vi "Main Loop.vi"(8 "error in (no error)":errorcluster, 10 "Chart Notifier":refnum<notifier>, 11 "Message Queues":T1) -> (0 "error out":errorcluster)   [LabVIEW 2018, in "Agitator Module.lvlib" / "Agitator Module Engine.lvlib"]
uses:
  Agitator Module Engine.lvlib
  Agitator Message Queues.ctl
  support/Message Queue/Message Cluster.ctl
  Feed Module/Controls/Agitator Module Display.ctl
  Feed Module/Controls/Agitator Module State Cluster.ctl
  Pump Module Folder/Measure Instrument/State Enum.ctl
  Feed Module/Controls/Agitator Module Config Cluster.ctl
  <vilib>/Utility/miscctls.llb/LVPoint32TypeDef.ctl
  Feed Module/Controls/Agitator Module Settings Cluster.ctl
  IKA EUROSTAR/IKA EUROSTAR Settings.ctl
  <vilib>/Platform/TimedLoop/XDataNode/timing_clust.ctl
  <vilib>/Platform/TimedLoop/XDataNode/nitl_modes.ctl
  <vilib>/Platform/TimedLoop/XDataNode/wakeup.ctl
  Tag VIs/Tag FGV Operation Enum.ctl
  support/Message Queue/Enqueue Message (Single).vi
  <vilib>/Platform/TimedLoop/XDataNode/XDataNode.xnode
  support/Message Queue/Message Queue.lvlib
  <vilib>/Platform/TimedLoop/XDataNode/XDNodeRunTimeDep.lvlib
  Agitator Module.lvlib
  Shared Variables/Dynamic Shared Variables.lvlib
  support/Support Library.lvlib
  Pump Module Folder/Measure Instrument/Pump Module Engine.lvlib
  IKA EUROSTAR/IKA EUROSTAR.lvlib
panel:
  out "Period (s) 2":dbl format="%_4g"
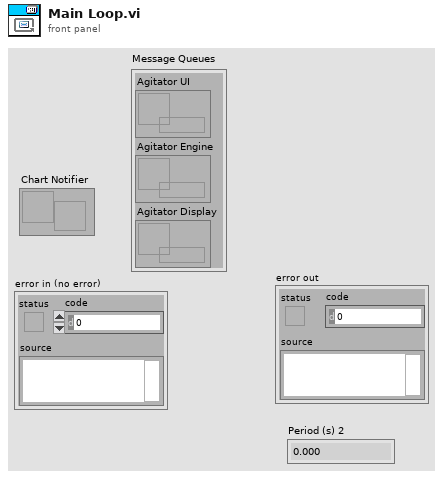
[diagram p1: front panel]
types:
  T1 = typedef "Agitator Module.lvlib/Agitator Message Queues.ctl" = cluster{"Agitator UI":refnum<queue>, "Agitator Engine":refnum<queue>, "Agitator Display":refnum<queue>}
  T2 = typedef "XDNodeRunTimeDep.lvlib/timing_clust.ctl" = cluster{"Expected End [f-1]":u64, "Actual End [f-1]":u64, "Finished Late? [f-1]":bool, "Expected End [i-1]":u64, "Actual End [i-1]":u64, "Finished Late? [i-1]":bool, "Expected Start [i]":u64, "Actual Start [i]":u64, "Expected Start [f]":u64, "Actual Start [f]":u64, "Source Name":string, "Structure Name":string, "Period":i64, "Deadline":i64, "Offset":i64, "Start":i64, "Priority":i32, "Timeout":i32, "Mode":T3, "Wakeup Reason":T4, "Error":errorcluster, "Source Type":string, "Secondary Source Type":string, "Global End Time":u64, "Global Start Time":u64, "Frame Duration":u64, "Iteration Duration":u64, "Assigned CPU":i32, "I/O Scan Engine Mode":u32}
  T3 = typedef "XDNodeRunTimeDep.lvlib/nitl_modes.ctl" = enum32{"No Change", "Process missed periods, maintain original phase", "Discard missed periods, maintain original phase", "Process missed periods, ignore original phase", "Discard missed periods, ignore original phase"}
  T4 = typedef "XDNodeRunTimeDep.lvlib/wakeup.ctl" = enum32{"Normal", "Aborted", "Asynchronous wakeup", "Timing source error", "Timed loop error", "Timeout"}
  T5 = cluster{"enable? (F)":bool, "name":string, "alarm on":bool, "priority":u32, "ack type":enum16{"Auto", "User", "None", "Each Occurrence"}, "area":string, "description":string, "log? (T)":bool}
  T6 = typedef "Tag FGV Operation Enum.ctl" = enum16{"Init", "Set Notification Queue", "Create Tag", "Commit", "Write Tag (Numeric)", "Write Tag (Boolean)", "Read All Tags", "Read One Tag", "Delete Tag Category", "Set Alarm Parameters (Numeric)", "Set Alarm Parameters (Boolean)", "Enable All Alarms", "Disable All Alarms", "Delete All Tags", "Read Alarms", "Ack Alarm", "Read Alarm Parameters (Numeric)", "Read Alarm Parameters (Boolean)"}
  T7 = enum32{"u32BitField", "bool", "double", "string", "int8", "uint8", "int16", "uint16", "int32", "uint32", "int64", "uint64", "single", "double waveform", "int16 waveform", "array of boolean", "array of int8", "array of uint8", "array of int16", "array of uint16", "array of int32", "array of uint32", "array of int64", "array of uint64", "array of single", "array of double", "array of double waveform", "array of int16 waveform", "array of string", "variant", "timestamp", "fixed point", "custom"}
  T8 = typedef "Pump Module.lvlib/Pump Module Engine.lvlib/State Enum.ctl" = enum16{"Measuring", "Idle", "Paused"}
  T9 = typedef "Agitator Module.lvlib/Agitator Module Config Cluster.ctl" = cluster{"GUID":string, "Drop Coords":T10, "Process Name":string, "User name":string, "Queue Name":string, "Settings":T11, "Load Count":i32}
  T10 = typedef "LVPoint32TypeDef.ctl" = cluster{"Horizontal":i32, "Vertical":i32}
  T11 = typedef "Agitator Module.lvlib/Agitator Module Settings Cluster.ctl" = cluster{"Cycle Period":dbl, "Agitator Type":string, "Setpoint (µm)":dbl, "IKA EUROSTAR Settings":T12}
  T12 = typedef "IKA EUROSTAR.lvlib/IKA EUROSTAR Settings.ctl" = cluster{"VISA resource name":refnum<visa-resource-name>, "Simulated?":bool}
  T13 = typedef "Agitator Module.lvlib/Agitator Module State Cluster.ctl" = cluster{"State":T8, "Start Time":timestamp, "Current Time":timestamp, "Agitator Module Config":T9, "Output Error":bool, "Log Started":bool, "First Iteration":bool, "Data":cluster{"Agitator rpm Value":dbl}, "Agitator On?":enum16{"Off", "On", "Not Initialized", "Over Cutoff"}}
  T14 = typedef "Agitator Module.lvlib/Agitator Module Display.ctl" = cluster{"Agitator On?":enum16{"Off", "On", "Not Initialized", "Over Cutoff"}, "Agitator RPM Value":dbl, "Cycle Period":dbl}
  T15 = enum16{"Off", "On", "Not Initialized", "Over Cutoff"}
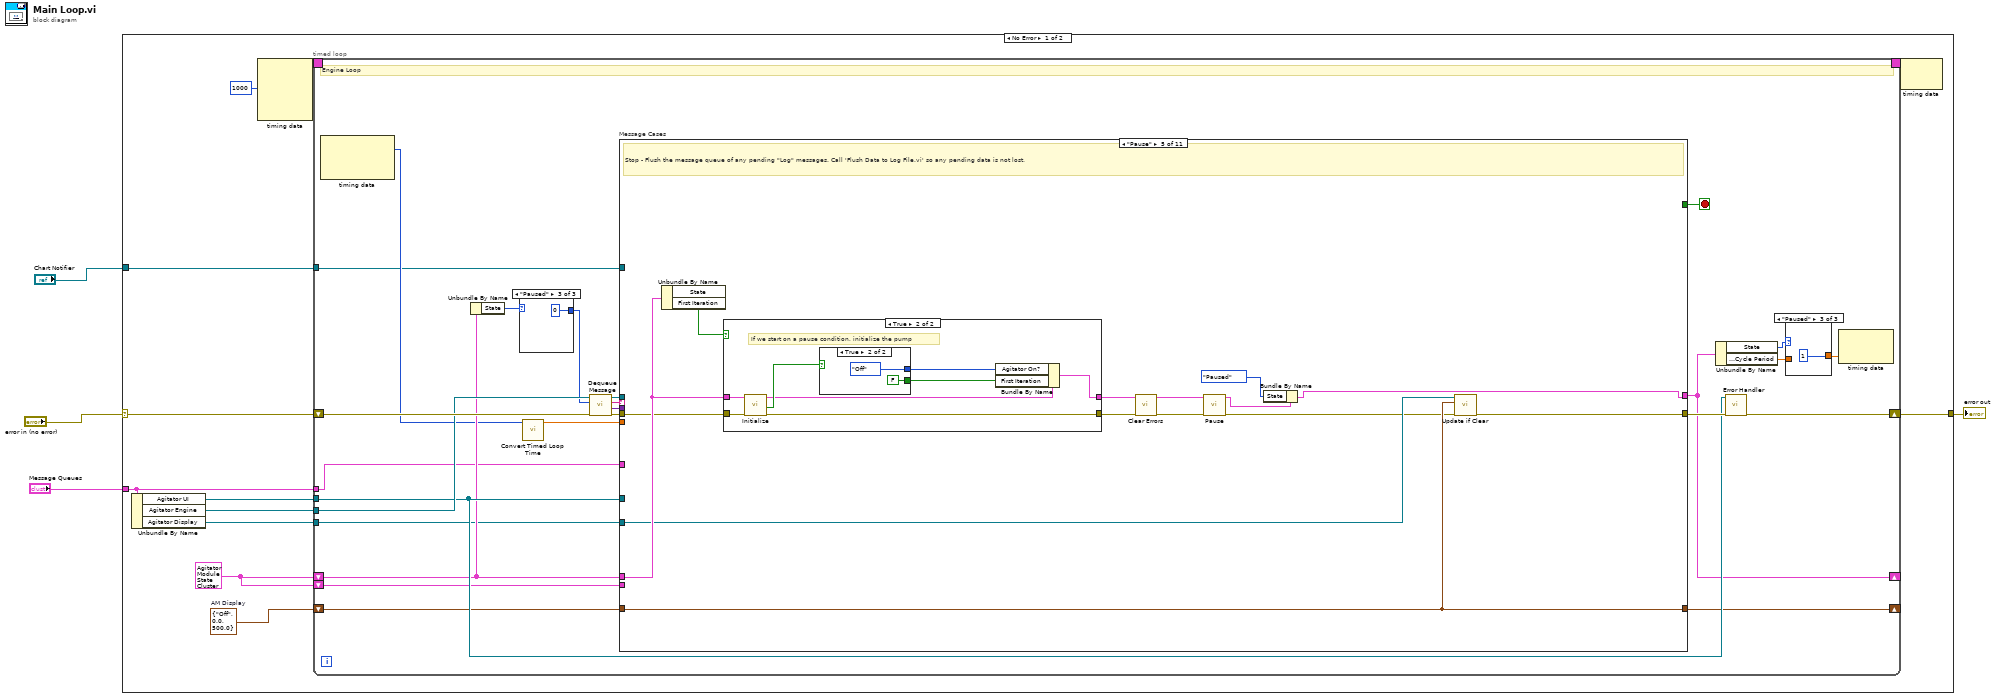
[diagram p0: block diagram]
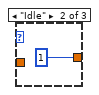
[diagram p3: hidden frame]
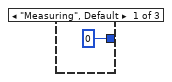
[diagram p4: hidden frame]
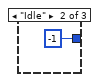
[diagram p5: hidden frame]
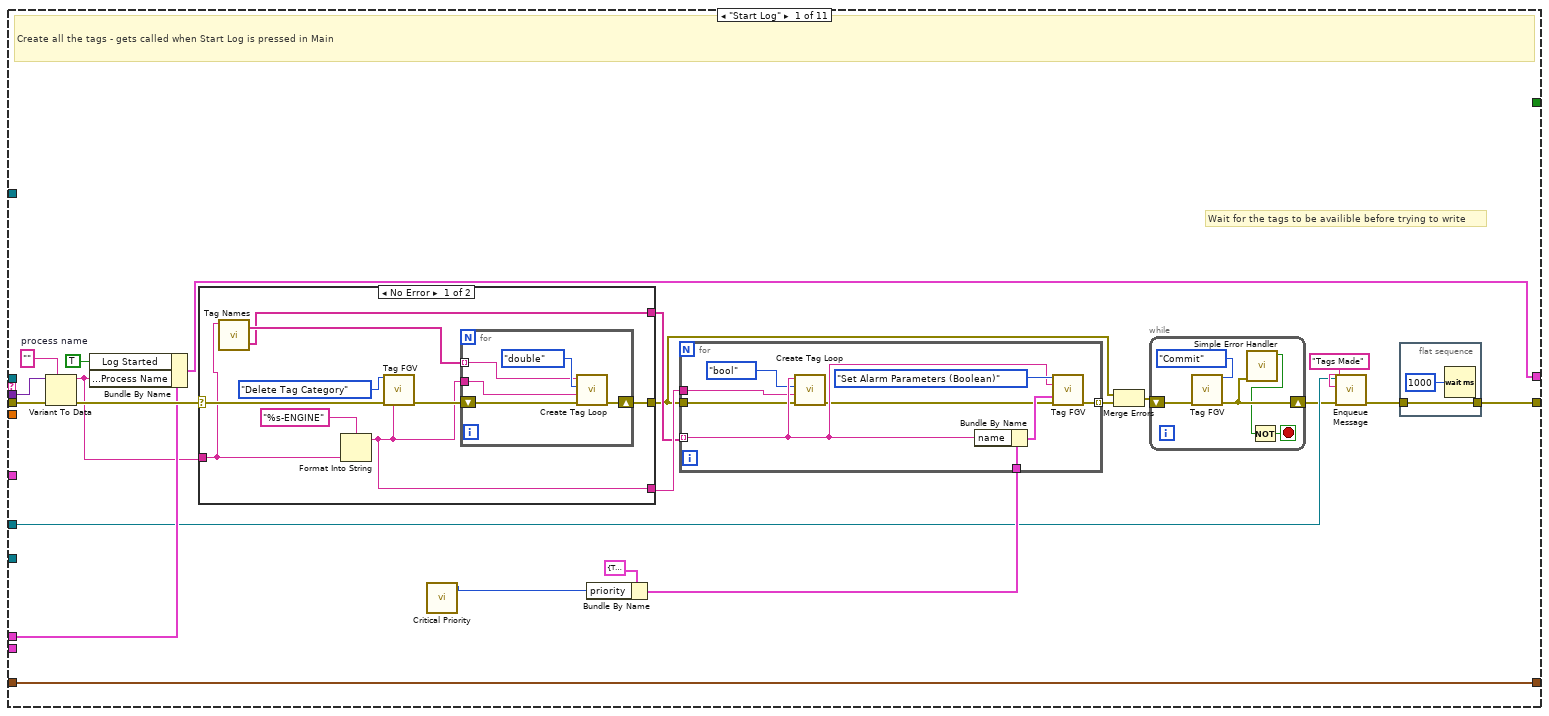
[diagram p6: hidden frame]
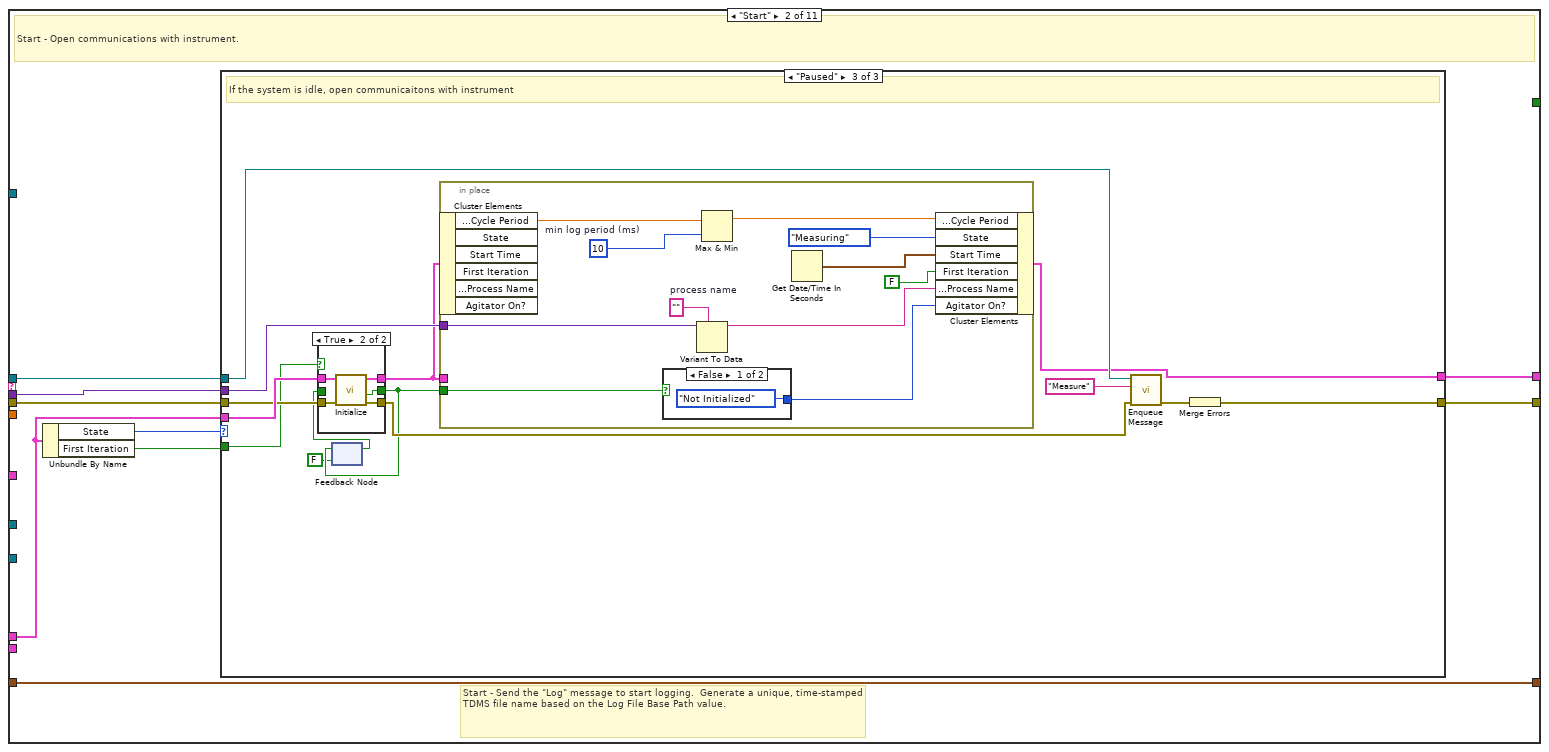
[diagram p8: hidden frame]
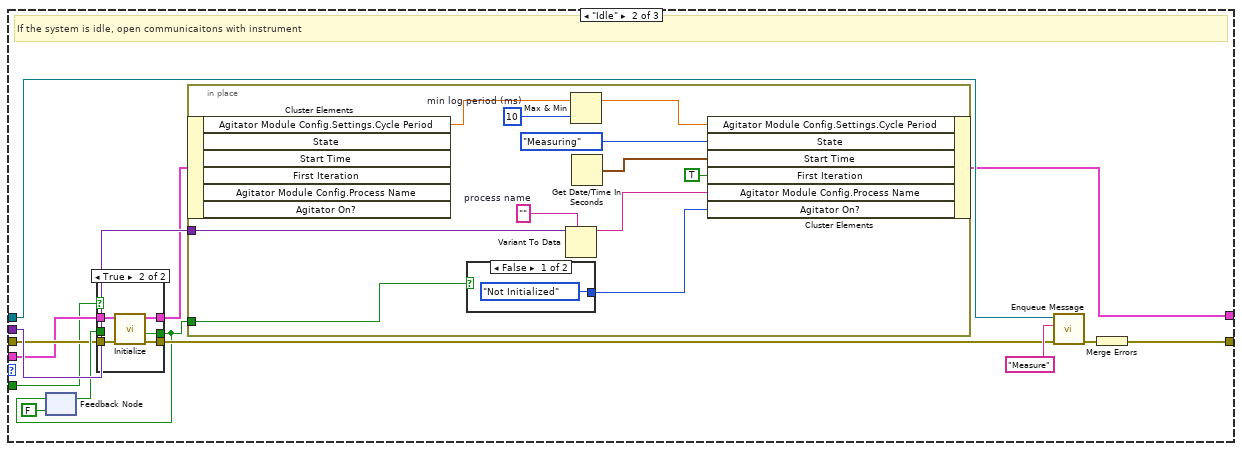
[diagram p10: hidden frame]
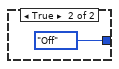
[diagram p11: hidden frame]
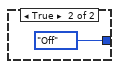
[diagram p13: hidden frame]
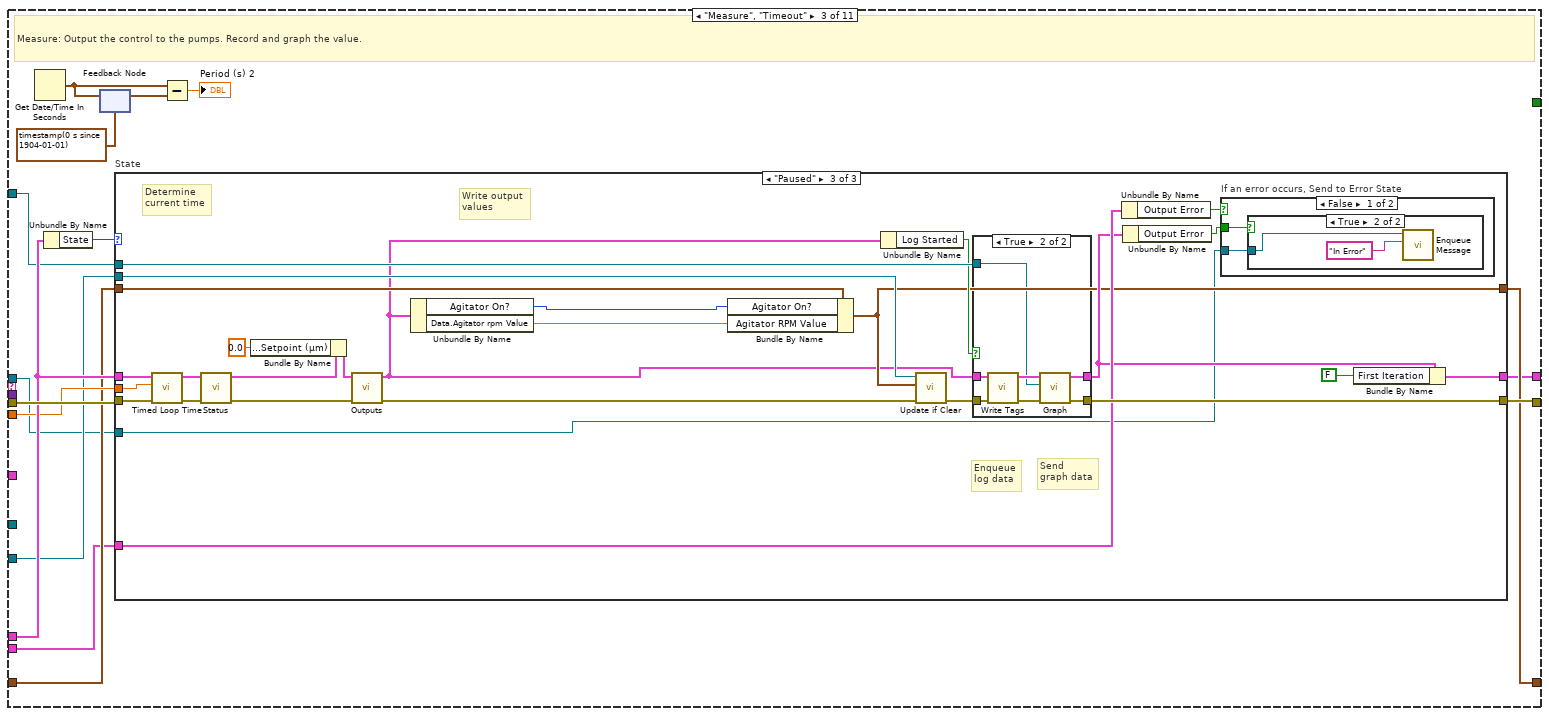
[diagram p15: hidden frame]
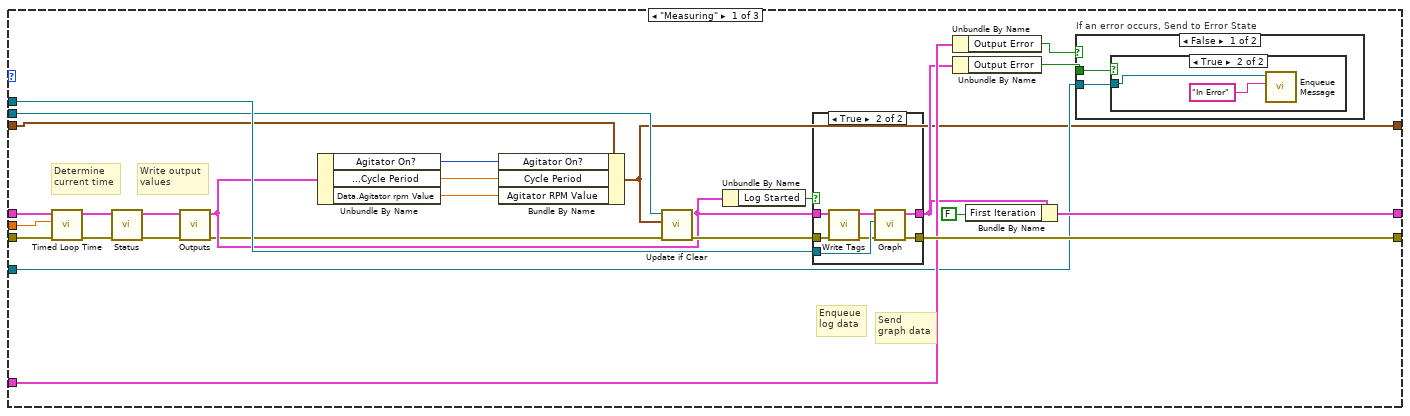
[diagram p16: hidden frame]
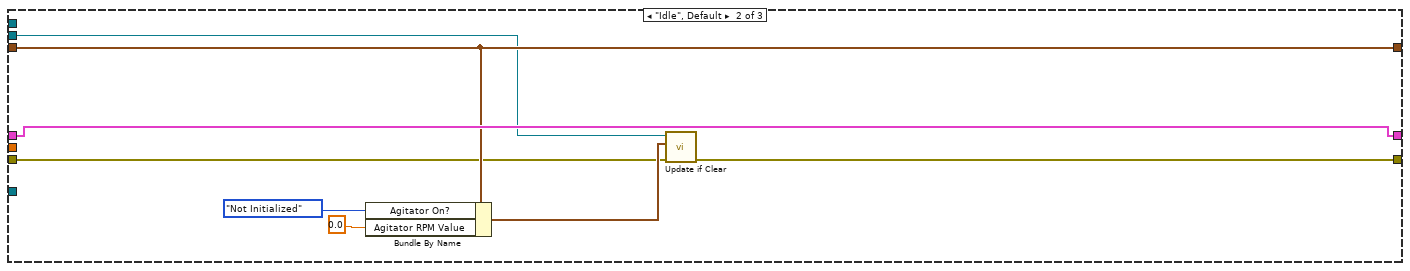
[diagram p20: hidden frame]
diagram:
  n1 = case shown="No Error" "error in (no error)" {
    selector: "error in (no error)" -> [w15 w405]
    tunnel: "Message Queues" -> [w11 _]
    tunnel: [w16 w405] -> w4
    tunnel: "Chart Notifier" -> [w9 _]
    frame No Error {
      w5 = T13 {"State"=enum."Idle", "Start Time"=timestamp(0 s since 1904-01-01), "Current Time"=timestamp(0 s since 1904-01-01), "Agitator Module Config"={"GUID"="", "Drop Coords"={"Horizontal"=0, "Vertical"=0}, "Process Name"="", "User name"="", "Queue Name"="", "Settings"={"Cycle Period"=500.0, "Agitator Type"="", "Setpoint (µm)"=0.0, "IKA EUROSTAR Settings"={"VISA resource name"="", "Simulated?"=FALSE}}, "Load Count"=0}, "Output Error"=FALSE, "Log Started"=FALSE, "First Iteration"=FALSE, "Data"={"Agitator rpm Value"=0.0}, "Agitator On?"=enum."Off"} ("Sonicator Module State Cluster")
      w6 = T14 {"Agitator On?"=enum."Off", "Agitator RPM Value"=0.0, "Cycle Period"=500.0}  # AM Display
      n2 = Unbundle By Name(w11) -> ("Agitator UI"=w14:refnum<queue>, "Agitator Engine"=w10:refnum<queue>, "Agitator Display"=w8:refnum<queue>)
      n3 = node-c288(i64 1000 ("Period")) -> (w13:T2)  [unwired: 3 in]
      n4 = timed-loop {
        tunnel: w10 -> [w35]
        shift-right: [w17] -> _
        shift-left: w5 -> [w31]
        shift-right: [w33] -> w16
        shift-left: w15 -> [w40]
        tunnel: w14 -> [w32]
        timing: w13 -> [_]
        timing-out: [_] -> w12
        tunnel: w11 -> [w23]
        tunnel: w9 -> [w22]
        tunnel: w8 -> [w21]
        shift-right: [w20] -> _
        shift-left: w6 -> [w19]
        shift-left: w5 -> [w18]
        stop <- w41 stop-if-true
        # "Engine Loop"
        n5 = node-c288() -> (w25:i64)  [unwired: 1 in, 2 out]
        n6 = Unbundle By Name(w31) -> ("State"=w30:T8)
        n7 = case shown="\"Paused\"" w30 {
          tunnel: [0 ("timeout in ms (-1)") -1 ("timeout in ms (-1)") 0 ("timeout in ms (-1)")] -> w29
          frame "Measuring", Default {
          }
          frame "Idle" {
          }
          frame "Paused" {
          }
        }
        n8 = call "Convert Timed Loop Time.vi"("Actual Start [i]"=w25) -> ("ET since start (s)"=w24:dbl)  [unwired: 10 in]
        n9 = call "Dequeue Message.vi"("error in (no error)"=w40, "timeout in ms (-1)"=w29, "Message Queue"=w35) -> ("error out"=w39:errorcluster, "Message Data"=w37:variant, "Message"=w38:string, "dup Message Queue"=w36:refnum<queue>)  [unwired: 5 in]
        n10 = case "Message Cases" shown="\"Pause\"" w38 {
          selector: w38 -> [_ _ _ _ _ _ _ _ _ _ w394]
          tunnel: w36 -> [_ w113 w190 _ _ _ w349 _ w368 _ _]
          tunnel: w39 -> [w59 w112 w200 w295 w321 w343 w352 w359 w363 w392 _]
          tunnel: [w55 w114 w201 w290 w318 w340 w354 w358 w373 w391 w393] -> w34
          tunnel: w31 -> [w64 w109 w199 w297 w322 w341 w345 w356 w364 w389 w399]
          tunnel: [w53 w106 w188 w296 w311 w339 w345 w356 w374 w387 w399] -> w17
          tunnel: [_ _ _ _ _ _ TRUE _ _ _ _] -> w41
          tunnel: w37 -> [w73 w110 _ _ _ w344 _ _ _ _ _]
          tunnel: w32 -> [w61 _ _ w299 _ _ w353 _ _ _ _]
          tunnel: w24 -> [_ _ w198 _ _ _ _ _ _ _ _]
          tunnel: w23 -> [_ _ _ _ _ _ _ _ _ _ _]
          tunnel: w22 -> [_ _ w194 _ _ _ _ _ _ _ _]
          tunnel: w21 -> [_ _ w193 w293 w320 _ _ _ w367 _ _]
          tunnel: w19 -> [w74 w108 w192 w292 w319 w342 w346 w357 w372 w390 w400]
          tunnel: [w74 w108 w191 w292 w319 w342 w346 w357 w366 w390 w400] -> w20
          tunnel: w18 -> [_ _ w189 _ _ _ _ _ _ _ _]
          frame "Start Log" {
            w72 = ""  # process name
            # "Wait for the tags to be availible before trying to write"
            # "Create all the tags - gets called when Start Log is pressed in Main"
            n11 = Variant To Data(error in=w59, type=w72, Variant=w73) -> (data=w60:string, error out=w71:errorcluster)
            n12 = Bundle By Name(cluster=w64, "Log Started"=TRUE, "Agitator Module Config.Process Name"=w60) -> (w53:T13)
            n13 = case shown="No Error" w71 {
              selector: w71 -> [w96 w105]
              tunnel: [w99 w105] -> w54
              tunnel: [w94 _] -> w67
              tunnel: [w92 _] -> w66
              tunnel: w60 -> [w91 _]
              frame No Error {
                n14 = call "Tag Names.vi"("Process Name"=w91) -> ("All Boolean Tags"=w92:string[], "All  Numeric Tags"=w93:string[])  [unwired: 8 in, 1 out]
                n15 = Format Into String(format string="%s-ENGINE", w91) -> (resulting string=w94:string)  [unwired: 2 in, 1 out]
                n16 = call "Tag FGV.vi"("Operation"=Tag_FGV_Operation_Enum."Delete Tag Category", "error in (no error)"=w96, "Tag Category"=w94) -> ("error out"=w95:errorcluster)  [unwired: 5 in, 7 out]
                n17 = for {
                  shift-right: [w100] -> w99
                  shift-left: w95 -> [w101]
                  tunnel: w94 -> [w102]
                  tunnel: w93 -> [w103] mode=indexing
                  n18 = call "Create Tag Loop.vi"("error in (no error)"=w101, "Tag Category"=w102, "data type"=T7."double", "Tag Name"=w103) -> ("error out"=w100:errorcluster)  [unwired: 7 in]
                }
              }
              frame Error {
              }
            }
            n19 = call "Critical Priority.vi"() -> ("critical priority"=w70:i32)  [unwired: 11 in]
            n20 = Bundle By Name(cluster=T5 {"enable? (F)"=TRUE, "name"="Boolean", "alarm on"=TRUE, "priority"=1, "ack type"=enum."Each Occurrence", "area"="a", "description"="", "log? (T)"=TRUE} ("Boolean alarm settings"), "priority"=w70) -> (w68:T5)
            n21 = for {
              tunnel: w68 -> [w90]
              tunnel: [w89] -> w65 mode=indexing
              tunnel: w66 -> [w86] mode=indexing
              tunnel: w54 -> [w83]
              tunnel: w67 -> [w84]
              n22 = call "Create Tag Loop.vi"("error in (no error)"=w83, "Tag Category"=w84, "data type"=T7."bool", "Tag Name"=w86) -> ("error out"=w82:errorcluster)  [unwired: 7 in]
              n23 = Bundle By Name(cluster=w90, "name"=w86) -> (w88:T5)
              n24 = call "Tag FGV.vi"("Operation"=Tag_FGV_Operation_Enum."Set Alarm Parameters (Boolean)", "Tag Name"=w86, "Data"=w88, "error in (no error)"=w82) -> ("error out"=w89:errorcluster)  [unwired: 4 in, 7 out]
            }
            n25 = Merge Errors(w54, w65) -> (w58:errorcluster)
            n26 = while {
              shift-right: [w79] -> w57
              shift-left: w58 -> [w80]
              stop <- w77 stop-if-true
              n27 = call "Tag FGV.vi"("Operation"=Tag_FGV_Operation_Enum."Commit", "error in (no error)"=w80) -> ("error out"=w79:errorcluster)  [unwired: 6 in, 7 out]
              n28 = call <vilib>:"Simple Error Handler.vi"("error in (no error)"=w79) -> ("error?"=w78:bool)  [unwired: 4 in, 4 out]
              n29 = Not(x=w78) -> (.not. x?=w77:bool)
            }
            n30 = call-poly "Enqueue Message.vi"("error in (no error)"=w57, "Message"="Tags Made", "Message Queue"=w61) -> ("error out"=w56:errorcluster)  [unwired: 7 in, 1 out]
            n31 = flat-sequence {
              tunnel: [w75] -> w55
              tunnel: w56 -> [w75]
              frame #0 {
                n32 = Wait (ms)(milliseconds to wait=u32 1000) -> ()  [unwired: 1 out]
              }
            }
          }
          frame "Start" {
            # "Start - Send the \"Log\" message to start logging.  Generate a unique, time-stamped TDMS file name based on the Log File Base Path value."
            # "Start - Open communications with instrument."
            n33 = Unbundle By Name(w109) -> ("State"=w111:T8, "First Iteration"=w107:bool)
            n34 = case shown="\"Paused\"" w111 {
              tunnel: [w115 w130 w165] -> w114
              tunnel: w113 -> [_ w127 w162]
              tunnel: w112 -> [w115 w124 w159]
              tunnel: w109 -> [w116 w123 w160]
              tunnel: [w116 w118 w153] -> w106
              tunnel: w110 -> [_ w126 w161]
              tunnel: w107 -> [_ w120 w155]
              frame "Measuring", Default {
                # "The system is already running. Ignore the \"Start\" message."
              }
              frame "Idle" {
                # "If the system is idle, open communicaitons with instrument"
                n35 = feedback #1(FALSE ("Initialized")) -> (w125:bool)
                n36 = case shown="True" w120 {
                  tunnel: w124 -> [w146 w147]
                  tunnel: w123 -> [w144 w148]
                  tunnel: [w144 w151] -> w119
                  tunnel: [w146 w150] -> w122
                  tunnel: [w145 w149] -> w121
                  tunnel: w125 -> [w145 _]
                  frame False {
                  }
                  frame True {
                    n37 = call "Initialize.vi"("error in (no error)"=w147, "Agitator Module State Cluster"=w148) -> ("error out"=w150:errorcluster, "Initialized"=w149:bool, "Agitator Module State Cluster"=w151:T13)  [unwired: 7 in]
                  }
                }
                n38 = feedback-in #1(w121) -> ()
                n39 = in-place {
                  in-place-border: w126 -> [w139]
                  in-place-border: w121 -> [w138]
                  w140 = ""  # process name
                  w141 = 10  # min log period (ms)
                  n40 = in-place-cluster #2(w119) -> ("Agitator Module Config.Settings.Cycle Period"=w137:dbl)  [unwired: 5 out]
                  n41 = case shown="False" w138 {
                    tunnel: [enum16{"Off", "On", "Not Initialized"}."Not Initialized" ("Pump On?") enum16{"Off", "On", "Not Initialized"}."Off" ("Pump On?")] -> w131
                    frame False {
                    }
                    frame True {
                    }
                  }
                  n42 = Variant To Data(type=w140, Variant=w139) -> (data=w132:string)  [unwired: 1 in, 1 out]
                  n43 = Max & Min(x=w137, y=w141) -> (max(x,y)=w136:dbl)  [unwired: 1 out]
                  n44 = Get Date/Time In Seconds() -> (seconds since 1Jan1904=w134:timestamp)
                  n45 = in-place-cluster #2("Agitator Module Config.Settings.Cycle Period"=w136, "State"=State_Enum."Measuring", "Start Time"=w134, "First Iteration"=TRUE, "Agitator Module Config.Process Name"=w132, "Agitator On?"=w131) -> (w118:T13)
                }
                n46 = call-poly "Enqueue Message.vi"("error in (no error)"=w122, "Message"="Measure", "Message Queue"=w127) -> ("error out"=w128:errorcluster)  [unwired: 7 in, 1 out]
                n47 = Merge Errors(w128) -> (w130:errorcluster)
              }
              frame "Paused" {
                # "If the system is idle, open communicaitons with instrument"
                n48 = feedback #3(FALSE ("Initialized")) -> (w156:bool)
                n49 = case shown="True" w155 {
                  tunnel: w159 -> [w180 w185]
                  tunnel: w160 -> [w181 w186]
                  tunnel: [w181 w182] -> w154
                  tunnel: [w180 w183] -> w158
                  tunnel: [w179 w184] -> w157
                  tunnel: w156 -> [w179 _]
                  frame False {
                  }
                  frame True {
                    n50 = call "Initialize.vi"("error in (no error)"=w185, "Agitator Module State Cluster"=w186) -> ("error out"=w183:errorcluster, "Initialized"=w184:bool, "Agitator Module State Cluster"=w182:T13)  [unwired: 7 in]
                  }
                }
                n51 = feedback-in #3(w157) -> ()
                n52 = in-place {
                  in-place-border: w161 -> [w174]
                  in-place-border: w154 -> [_]
                  in-place-border: w157 -> [w173]
                  w175 = ""  # process name
                  w176 = 10  # min log period (ms)
                  n53 = in-place-cluster #4(w154) -> ("Agitator Module Config.Settings.Cycle Period"=w172:dbl)  [unwired: 5 out]
                  n54 = case shown="False" w173 {
                    tunnel: [enum16{"Off", "On", "Not Initialized"}."Not Initialized" ("Pump On?") enum16{"Off", "On", "Not Initialized"}."Off" ("Pump On?")] -> w166
                    frame False {
                    }
                    frame True {
                    }
                  }
                  n55 = Variant To Data(type=w175, Variant=w174) -> (data=w167:string)  [unwired: 1 in, 1 out]
                  n56 = Max & Min(x=w172, y=w176) -> (max(x,y)=w171:dbl)  [unwired: 1 out]
                  n57 = Get Date/Time In Seconds() -> (seconds since 1Jan1904=w169:timestamp)
                  n58 = in-place-cluster #4("Agitator Module Config.Settings.Cycle Period"=w171, "State"=State_Enum."Measuring", "Start Time"=w169, "First Iteration"=FALSE, "Agitator Module Config.Process Name"=w167, "Agitator On?"=w166) -> (w153:T13)
                }
                n59 = call-poly "Enqueue Message.vi"("error in (no error)"=w158, "Message"="Measure", "Message Queue"=w162) -> ("error out"=w163:errorcluster)  [unwired: 7 in, 1 out]
                n60 = Merge Errors(w163) -> (w165:errorcluster)
              }
            }
          }
          frame "Measure", "Timeout" {
            # "Measure: Output the control to the pumps. Record and graph the value."
            n61 = Get Date/Time In Seconds() -> (seconds since 1Jan1904=w196:timestamp)
            n62 = Unbundle By Name(w199) -> ("State"=w202:T8)
            n63 = feedback-in #5(w196) -> ()
            n64 = feedback #5(timestamp(0 s since 1904-01-01) ("seconds since 1Jan1904")) -> (w197:timestamp)
            n65 = case "State" shown="\"Paused\"" w202 {
              tunnel: w200 -> [w210 w243 w260]
              tunnel: w199 -> [w211 w249 w261]
              tunnel: [w228 w242 w273] -> w201
              tunnel: [w227 w249 w267] -> w188
              tunnel: w198 -> [w209 _ w262]
              tunnel: w194 -> [w225 _ w276]
              tunnel: w193 -> [w214 w245 w265]
              tunnel: w192 -> [w224 w248 w275]
              tunnel: [w213 w248 w264] -> w191
              tunnel: w190 -> [w215 _ w251]
              tunnel: w189 -> [w217 _ w271]
              frame "Measuring" {
                # "Determine\ncurrent time"
                # "Send\ngraph data"
                # "Enqueue\nlog data"
                # "Write output\nvalues"
                n66 = call "Timed Loop Time.vi"("error in (no error)"=w210, "ET since start (s)"=w209, "Agitator Module State Cluster"=w211) -> ("error out"=w207:errorcluster, "Agitator Module State Cluster"=w208:T13)  [unwired: 7 in]
                n67 = call "Status.vi"("error in (no error)"=w207, "Agitator Module State Cluster"=w208) -> ("error out"=w205:errorcluster, "Agitator Module State Cluster"=w206:T13)  [unwired: 8 in]
                n68 = call "Outputs.vi"("error in (no error)"=w205, "Agitator Module State Cluster"=w206) -> ("error out"=w203:errorcluster, "Agitator Module State Cluster"=w204:T13)  [unwired: 8 in]
                n69 = Unbundle By Name(w204) -> ("Agitator On?"=w223:T15, "Agitator Module Config.Settings.Cycle Period"=w222:dbl, "Data.Agitator rpm Value"=w221:dbl)
                n70 = Bundle By Name(cluster=w224, "Agitator On?"=w223, "Cycle Period"=w222, "Agitator RPM Value"=w221) -> (w213:T14)
                n71 = call "Update if Clear.vi"("error in (no error)"=w203, "Message Data"=w213, "Queue in"=w214) -> ("error out"=w212:errorcluster)  [unwired: 8 in]
                n72 = Unbundle By Name(w204) -> ("Log Started"=w220:bool)
                n73 = case shown="True" w220 {
                  tunnel: [w233 w236] -> w228
                  tunnel: [w234 w235] -> w216
                  tunnel: w225 -> [_ w239]
                  tunnel: w204 -> [w234 w241]
                  tunnel: w212 -> [w233 w237]
                  frame False {
                  }
                  frame True {
                    n74 = call "Write Tags.vi"("error in (no error)"=w237, "Agitator Module State Cluster"=w241) -> ("error out"=w238:errorcluster, "Agitator Module State Cluster"=w240:T13)  [unwired: 8 in]
                    n75 = call "Graph.vi"("error in (no error)"=w238, "notifier out"=w239, "Agitator Module State Cluster"=w240) -> ("error out"=w236:errorcluster, "Agitator Module State Cluster"=w235:T13)  [unwired: 7 in]
                  }
                }
                n76 = Unbundle By Name(w217) -> ("Output Error"=w218:bool)
                n77 = Unbundle By Name(w216) -> ("Output Error"=w219:bool)
                n78 = Bundle By Name(cluster=w216, "First Iteration"=FALSE) -> (w227:T13)
                n79 = case "If an error occurs, Send to Error State" shown="False" w218 {
                  tunnel: w219 -> [w230 _]
                  tunnel: w215 -> [w229 _]
                  frame False {
                    n80 = case shown="True" w230 {
                      tunnel: w229 -> [_ w231]
                      frame False {
                      }
                      frame True {
                        n81 = call-poly "Enqueue Message.vi"("Message"="In Error", "Message Queue"=w231) -> ()  [unwired: 8 in, 2 out]
                      }
                    }
                  }
                  frame True {
                  }
                }
              }
              frame "Idle", Default {
                n82 = Bundle By Name(cluster=w248, "Agitator On?"=enum16{"Off", "On", "Not Initialized"}."Not Initialized" ("Pump On?"), "Agitator RPM Value"=0.0 ("Current Pump Speed")) -> (w244:T14)
                n83 = call "Update if Clear.vi"("error in (no error)"=w243, "Message Data"=w244, "Queue in"=w245) -> ("error out"=w242:errorcluster)  [unwired: 8 in]
              }
              frame "Paused" {
                # "Determine\ncurrent time"
                # "Write output\nvalues"
                # "Send\ngraph data"
                # "Enqueue\nlog data"
                n84 = call "Timed Loop Time.vi"("error in (no error)"=w260, "ET since start (s)"=w262, "Agitator Module State Cluster"=w261) -> ("error out"=w258:errorcluster, "Agitator Module State Cluster"=w257:T13)  [unwired: 7 in]
                n85 = call "Status.vi"("error in (no error)"=w258, "Agitator Module State Cluster"=w257) -> ("error out"=w255:errorcluster, "Agitator Module State Cluster"=w259:T13)  [unwired: 8 in]
                n86 = Bundle By Name(cluster=w259, "Agitator Module Config.Settings.Setpoint (µm)"=0.0 ("Configuration.Manual Entry")) -> (w256:T13)
                n87 = call "Outputs.vi"("error in (no error)"=w255, "Agitator Module State Cluster"=w256) -> ("error out"=w254:errorcluster, "Agitator Module State Cluster"=w253:T13)  [unwired: 8 in]
                n88 = Unbundle By Name(w253) -> ("Agitator On?"=w250:T15, "Data.Agitator rpm Value"=w252:dbl)
                n89 = Bundle By Name(cluster=w275, "Agitator On?"=w250, "Agitator RPM Value"=w252) -> (w264:T14)
                n90 = Unbundle By Name(w253) -> ("Log Started"=w266:bool)
                n91 = call "Update if Clear.vi"("error in (no error)"=w254, "Message Data"=w264, "Queue in"=w265) -> ("error out"=w263:errorcluster)  [unwired: 8 in]
                n92 = case shown="True" w266 {
                  tunnel: w276 -> [_ w282]
                  tunnel: w263 -> [w278 w285]
                  tunnel: [w278 w280] -> w273
                  tunnel: [w277 w279] -> w268
                  tunnel: w253 -> [w277 w284]
                  frame False {
                  }
                  frame True {
                    n93 = call "Write Tags.vi"("error in (no error)"=w285, "Agitator Module State Cluster"=w284) -> ("error out"=w281:errorcluster, "Agitator Module State Cluster"=w283:T13)  [unwired: 8 in]
                    n94 = call "Graph.vi"("error in (no error)"=w281, "notifier out"=w282, "Agitator Module State Cluster"=w283) -> ("error out"=w280:errorcluster, "Agitator Module State Cluster"=w279:T13)  [unwired: 7 in]
                  }
                }
                n95 = Unbundle By Name(w271) -> ("Output Error"=w270:bool)
                n96 = Unbundle By Name(w268) -> ("Output Error"=w272:bool)
                n97 = case "If an error occurs, Send to Error State" shown="False" w270 {
                  tunnel: w272 -> [w287 _]
                  tunnel: w251 -> [w286 _]
                  frame False {
                    n98 = case shown="True" w287 {
                      tunnel: w286 -> [_ w289]
                      frame False {
                      }
                      frame True {
                        n99 = call-poly "Enqueue Message.vi"("Message"="In Error", "Message Queue"=w289) -> ()  [unwired: 8 in, 2 out]
                      }
                    }
                  }
                  frame True {
                  }
                }
                n100 = Bundle By Name(cluster=w268, "First Iteration"=FALSE) -> (w267:T13)
              }
            }
            n101 = Subtract(x=w196, y=w197) -> (x-y=→"Period (s) 2":dbl)
          }
          frame "Stop" {
            # "Stop - Flush the message queue of any pending \"Log\" messages. Call 'Flush Data to Log File.vi' so any pending data is not lost."
            n102 = call <vilib>:"Clear Errors.vi"("error in (no error)"=w295) -> ("error out"=w294:errorcluster)  [unwired: 5 in, 1 out]
            n103 = Unbundle By Name(w297) -> ("State"=w298:T8)
            n104 = case shown="\"Measuring\", Default" w298 {
              tunnel: [w304 w310] -> w291
              tunnel: w294 -> [w302 w310]
              tunnel: w299 -> [w308 _]
              tunnel: w297 -> [w303 w309]
              tunnel: [w306 w309] -> w296
              frame "Measuring", Default {
                # "If the system is logging, stop logging."
                n105 = call "Close.vi"("error in (no error)"=w302, "Agitator Module State Cluster"=w303) -> ("error out"=w300:errorcluster, "Agitator Module State Cluster"=w301:T13)  [unwired: 8 in]
                n106 = Bundle By Name(cluster=w301, "State"=State_Enum."Idle") -> (w306:T13)
                n107 = call-poly "Enqueue Message.vi"("error in (no error)"=w300, "Message"="Logging Stopped", "Message Queue"=w308) -> ("error out"=w304:errorcluster)  [unwired: 7 in, 1 out]
              }
              frame "Idle" {
                # "The system is already idle. Ignore the \"Stop\" message."
              }
            }
            n108 = call "Update if Clear.vi"("error in (no error)"=w291, "Message Data"=w292, "Queue in"=w293) -> ("error out"=w290:errorcluster)  [unwired: 8 in]
          }
          frame "Pause" {
            # "Stop - Flush the message queue of any pending \"Log\" messages. Call 'Flush Data to Log File.vi' so any pending data is not lost."
            n109 = Unbundle By Name(w322) -> ("First Iteration"=w323:bool)  [unwired: 1 out]
            n110 = case shown="True" w323 {
              tunnel: w322 -> [w324 w330]
              tunnel: [w324 w332] -> w315
              tunnel: w321 -> [w325 w326]
              tunnel: [w325 w327] -> w316
              frame False {
              }
              frame True {
                # "If we start on a pause condition, initialize the pump"
                n111 = call "Initialize.vi"("error in (no error)"=w326, "Agitator Module State Cluster"=w330) -> ("error out"=w327:errorcluster, "Initialized"=w329:bool, "Agitator Module State Cluster"=w328:T13)  [unwired: 7 in]
                n112 = case shown="True" w329 {
                  tunnel: [enum16{"Off", "On", "Not Initialized"}."Not Initialized" ("Pump On?") enum16{"Off", "On", "Not Initialized"}."Off" ("Pump On?")] -> w333
                  tunnel: [_ FALSE] -> w331
                  frame False {
                  }
                  frame True {
                  }
                }
                n113 = Bundle By Name(cluster=w328, "Agitator On?"=w333, "First Iteration"=w331) -> (w332:T13)
              }
            }
            n114 = call <vilib>:"Clear Errors.vi"("error in (no error)"=w316) -> ("error out"=w314:errorcluster)  [unwired: 5 in, 1 out]
            n115 = call "Pause.vi"("error in (no error)"=w314, "Sonicator Module State Cluster"=w315) -> ("error out"=w312:errorcluster, "Sonicator Module State Cluster"=w313:T13)  [unwired: 8 in]
            n116 = Bundle By Name(cluster=w313, "State"=State_Enum."Paused") -> (w311:T13)
            n117 = call "Update if Clear.vi"("error in (no error)"=w312, "Message Data"=w319, "Queue in"=w320) -> ("error out"=w318:errorcluster)  [unwired: 8 in]
          }
          frame "Update Settings" {
            # "New settings are available, update the current ones stored in the shift register with the settings sent as part of the message"
            n118 = Variant To Data(error in=w343, type=T9 {"GUID"="", "Drop Coords"={"Horizontal"=0, "Vertical"=0}, "Process Name"="", "User name"="", "Queue Name"="", "Settings"={"Cycle Period"=500.0, "Agitator Type"="", "Setpoint (µm)"=0.0, "IKA EUROSTAR Settings"={"VISA resource name"="", "Simulated?"=FALSE}}, "Load Count"=0} ("Sonicator Module Config"), Variant=w344) -> (data=w338:T9, error out=w340:errorcluster)
            n119 = Bundle By Name(cluster=w341, "Agitator Module Config"=w338) -> (w339:T13)
          }
          frame "Exit" {
            # "Release the Logging queue reference"
            # "Don't check the error out. The UI message queue may have already been released."
            # "Stop the VI"
            # "Exit - Send the Exit message to the UI Message Handler.  Call 'Flush Data to Log File.vi' so any pending data is not lost."
            n120 = Release Queue(queue=w349, error in (no error)=w352) -> (error out=w348:errorcluster)  [unwired: 1 in, 2 out]
            n121 = call-poly "Enqueue Message.vi"("Priority Message? (F)"=TRUE, "Message"="Exit", "Message Queue"=w353) -> ("error out"=w347:errorcluster)  [unwired: 7 in, 1 out]
            n122 = call <vilib>:"Clear Errors.vi"("error in (no error)"=w347) -> ()  [unwired: 5 in, 2 out]
            n123 = Merge Errors(w348) -> (w354:errorcluster)
          }
          frame "---Copy This Frame---" {
            # "Duplicate this frame when creating new messages.  Change this comment in the duplicated frame to describe this message."
            n124 = Merge Errors(w359) -> (w358:errorcluster)
          }
          frame "In Error" {
            # "If we have a disconnect Error we will go to this state, and attempt to reconnect and get back to the pre-error state"
            n125 = Merge Errors(w363) -> ()  [unwired: 1 out]
            n126 = call "Initialize.vi"("error in (no error)"=w363, "Agitator Module State Cluster"=w364) -> ("error out"=w361:errorcluster, "Initialized"=w360:bool, "Agitator Module State Cluster"=w362:T13)  [unwired: 7 in]
            n127 = Unbundle By Name(w362) -> ("Agitator On?"=w369:T15, "Agitator Module Config.Settings.Cycle Period"=w370:dbl, "Data.Agitator rpm Value"=w371:dbl)
            n128 = Bundle By Name(cluster=w372, "Agitator On?"=w369, "Cycle Period"=w370, "Agitator RPM Value"=w371) -> (w366:T14)
            n129 = call "Update if Clear.vi"("error in (no error)"=w361, "Message Data"=w366, "Queue in"=w367) -> ("error out"=w365:errorcluster)  [unwired: 8 in]
            n130 = case shown="False" w360 {
              tunnel: w368 -> [w379 w383]
              tunnel: w365 -> [w378 w382]
              tunnel: [w376 w385] -> w374
              tunnel: w362 -> [w376 w385]
              tunnel: [w375 w381] -> w373
              frame False {
                n131 = Wait (ms)(milliseconds to wait=u32 5000) -> ()  [unwired: 1 out]
                n132 = call-poly "Enqueue Message.vi"("error in (no error)"=w378, "Message"="In Error", "Message Queue"=w379) -> ("error out"=w375:errorcluster)  [unwired: 7 in, 1 out]
              }
              frame True {
                n133 = call-poly "Enqueue Message.vi"("error in (no error)"=w382, "Message"="Measure", "Message Queue"=w383) -> ("error out"=w381:errorcluster)  [unwired: 7 in, 1 out]
              }
            }
          }
          frame "Initialize" {
            # "Duplicate this frame when creating new messages.  Change this comment in the duplicated frame to describe this message."
            n134 = Merge Errors(w392) -> (w391:errorcluster)
            n135 = Bundle By Name(cluster=w389, "Log Started"=FALSE, "First Iteration"=TRUE) -> (w387:T13)
          }
          frame Default {
            # "'Default' case only runs if there is a message that isn't defined in any of the other cases.  Output a programming error."
            n136 = Concatenate Strings("The invalid message string " ("string"), w394, " was received in the Pump Module Engine." ("string")) -> (w395:string)
            n137 = Bundle By Name(cluster=errorcluster {"status"=TRUE, "code"=1, "source"=""} ("error constant"), "source"=w395) -> (w393:errorcluster)
          }
        }
        n138 = Unbundle By Name(w17) -> ("State"=w28:T8, "Agitator Module Config.Settings.Cycle Period"=w26:dbl)
        n139 = call "Error Handler.vi"("error in (no error)"=w34, "Message Queue"=w32) -> ("dup error in"=w33:errorcluster)  [unwired: 8 in, 1 out]
        n140 = case shown="\"Paused\"" w28 {
          tunnel: [w42 1 1] -> w27
          tunnel: w26 -> [w42 _ _]
          frame "Measuring" {
          }
          frame "Idle" {
          }
          frame "Paused" {
          }
        }
        n141 = node-c288(w27) -> ()  [unwired: 1 in, 1 out]
      }
      n142 = node-c288(w12) -> ()  [unwired: 1 out]
    }
    frame Error {
    }
  }
  "error out" <- w4
